vi "Add Parameter.vi"(8 "error in":errorcluster, 9 "parameter definition":T1={"start index"=0, "size"=8, "encoding"=enum."BCD", "signed"=FALSE, "scale multiplier"=1.0, "scale offset"=0.0}, 10 "parameter":T4, 11 "label ref":T3 format="%.0x") -> (0 "error out":errorcluster, 2 "parameter ref":T3 format="%.0x", 3 "label ref out":T3 format="%.0x")   [LabVIEW 2020, in "ARINC 429 Scripting.lvlib"]
uses:
  ARINC 429 Scripting.lvlib
  <vilib>/NI VeriStand/Custom Device API/Custom Device Item Ref.ctl
  Shared/Parameter Definition.ctl
  Encoding and Decoding/Encoding.ctl
  <vilib>/NI VeriStand/Custom Device API/Custom Device Channel.ctl
  <vilib>/NI VeriStand/Custom Device API/Custom Device Channel Type.ctl
  Ballard/Constants.vi
  <vilib>/NI VeriStand/Custom Device Tools/Custom Device Utility Library/NI VeriStand - Search for Item by GUID.vi
  Ballard/Ballard ARINC 429 Scripting.lvlib
  <vilib>/NI VeriStand/Custom Device API/Custom Device API.lvlib
  <vilib>/NI VeriStand/Custom Device Tools/Custom Device Utility Library/Custom Device Utility Library.lvlib
  Encoding and Decoding/Encoding and Decoding.lvlib
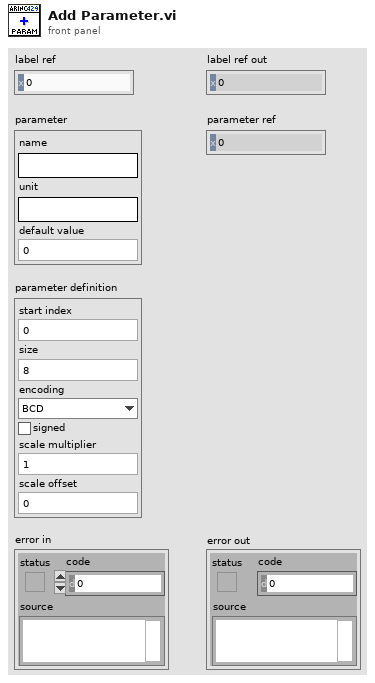
[diagram p1: front panel]
types:
  T1 = typedef "Parameter Definition.ctl" = cluster{"start index":i32, "size":i32, "encoding":T2, "signed":bool, "scale multiplier":dbl, "scale offset":dbl}
  T2 = typedef "Encoding and Decoding.lvlib/Encoding.ctl" = enum16{"BNR", "BCD", "Discrete"}
  T3 = typedef "Custom Device API.lvlib/Custom Device Item Ref.ctl" = u64
  T4 = cluster{"name":string, "unit":string, "default value":dbl}
  T5 = typedef "Custom Device API.lvlib/Custom Device Channel.ctl" = cluster{"Type":T6, "Units":string, "Default Value":dbl, "Faultable":bool, "Scalable":bool}
  T6 = typedef "Custom Device API.lvlib/Custom Device Channel Type.ctl" = enum16{"Input", "Output"}
  T7 = typedef "Direction.ctl" = enum16{"Rx", "Tx"}
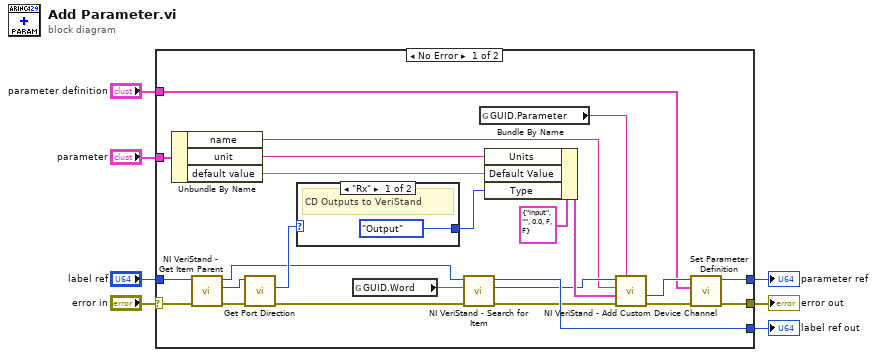
[diagram p0: block diagram]
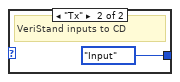
[diagram p2: hidden frame]
diagram:
  n1 = case shown="No Error" "error in" {
    selector: "error in" -> [w17 w35]
    tunnel: [w22 w35] -> w6
    tunnel: "label ref" -> [w16 w34]
    tunnel: [w23 _] -> w4
    tunnel: "parameter" -> [w27 _]
    tunnel: [w20 w34] -> w2
    tunnel: "parameter definition" -> [w8 _]
    frame No Error {
      n2 = Unbundle By Name(w27) -> ("name"=w11:string, "unit"=w28:string, "default value"=w26:dbl)
      n3 = call <vilib>:"NI VeriStand - Get Item Parent.vi"("error in (no error)"=w17, "Item Ref in"=w16) -> ("error out"=w15:errorcluster, "Parent Ref"=w10:T3, "Item Ref out"=w9:T3)  [unwired: 6 in, 1 out]
      n4 = call "Get Port Direction.vi"("error in"=w15, "port ref in"=w10) -> ("error out"=w14:errorcluster, "direction"=w13:T7)  [unwired: 7 in, 1 out]
      n5 = case shown="\"Rx\"" w13 {
        tunnel: [Custom_Device_Channel_Type."Output" ("Type") Custom_Device_Channel_Type."Input" ("Type")] -> w12
        frame "Rx" {
          # "CD Outputs to VeriStand"
        }
        frame "Tx" {
          # "VeriStand inputs to CD"
        }
      }
      n6 = global read "Constants.vi" "GUID.Word"() -> (w21:string)
      n7 = call-poly <vilib>:"NI VeriStand - Search for Item.vi"("error in"=w14, "Item GUID"=w21, "Section Ref in"=w9) -> ("error out"=w19:errorcluster, "Item Ref"=w18:T3, "Section Ref out"=w20:T3)  [unwired: 5 in, 1 out]
      n8 = global read "Constants.vi" "GUID.Parameter"() -> (w31:string)
      n9 = Bundle By Name(cluster=T5 {"Type"=enum."Input", "Units"="", "Default Value"=0.0, "Faultable"=FALSE, "Scalable"=FALSE} ("Channel"), "Units"=w28, "Default Value"=w26, "Type"=w12) -> (w29:T5)
      n10 = call <vilib>:"NI VeriStand - Add Custom Device Channel.vi"("GUID (Default Channel)"=w31, "error in (no error)"=w19, "Channel"=w29, "Channel Name"=w11, "Parent Ref in"=w18) -> ("error out"=w25:errorcluster, "Channel Ref"=w24:T3)  [unwired: 3 in, 2 out]
      n11 = call "Set Parameter Definition.vi"("error in"=w25, "parameter definition"=w8, "parameter ref in"=w24) -> ("error out"=w22:errorcluster, "parameter ref out"=w23:T3)  [unwired: 7 in]
    }
    frame Error {
    }
  }
  "parameter ref" <- w4
  "error out" <- w6
  "label ref out" <- w2
